vi "Resize Rendez-Vous.vi"(8 "error in (no error)":errorcluster, 10 "Resize":i32, 11 "SMO":refnum<class "SMO.lvclass">) -> (0 "error out":errorcluster, 3 "SMO out":refnum<class "SMO.lvclass">)   [LabVIEW 2013, in "SMO.lvclass"]
uses:
  SMO.lvclass
  SMO.lvclass/SMO.ctl
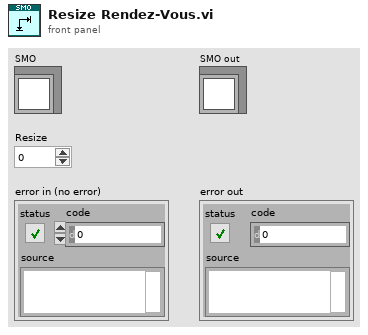
[diagram p1: front panel]
types:
  T1 = typedef "SMO.lvclass/PrivateData--Ref.ctl" = refnum<data-value>
  T2 = typedef "SMO.lvclass/PrivateData--Cluster.ctl" = cluster{"SMO Name":string, "Parent Call":T3, "Registered Processes":T4[], "Process Sync RendezVous":T5, "Process Error Notifier":refnum<notifier>, "Protected Events":T6, "Public Events":T7}
  T3 = typedef "SMO.lvclass/Parent Call--Enum.ctl" = enum16{"Allows parent to run", "Does not request parent to run"}
  T4 = typedef "SMO.lvclass/RegisteredProcessData--Cluster.ctl" = cluster{"Name":string, "Static VI Ref":refnum<vi>, "Running":bool}
  T5 = typedef "Rendezvous RefNum" = refnum<k1>
  T6 = typedef "SMO.lvclass/Protected Events.ctl" = cluster{"StopProcesses":refnum<user-event>, "AbortProcesses":refnum<user-event>}
  T7 = typedef "SMO.lvclass/Public Events.ctl" = cluster{"Error":refnum<user-event>}
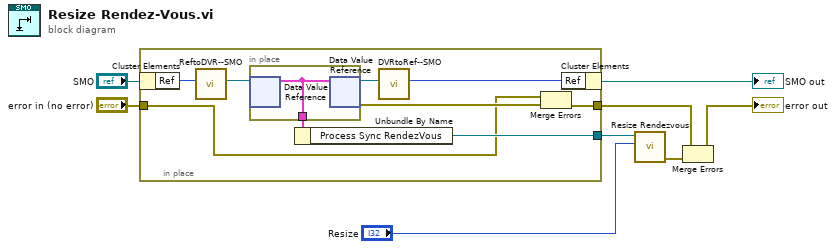
[diagram p0: block diagram]
diagram:
  n1 = in-place {
    in-place-border: [w15] -> w3
    in-place-border: [w10] -> w6
    in-place-border: "error in (no error)" -> [w9]
    n2 = in-place-cluster #1("SMO") -> ("Ref"=w14:u32)
    n3 = call "ReftoDVR--SMO.vi"("Ref"=w14) -> ("Ref"=w13:T1)  [unwired: 10 in]
    n4 = in-place {
      in-place-border: [w18] -> w17
      n5 = in-place-dvr #2(w13) -> (w18:T2)  [unwired: 1 out]
      n6 = in-place-dvr #2(w18) -> (w12:T1, w16:errorcluster)
    }
    n7 = Unbundle By Name(w17) -> ("Process Sync RendezVous"=w10:T5)
    n8 = call "DVRtoRef--SMO.vi"("Ref"=w12) -> ("Ref"=w11:u32)  [unwired: 10 in]
    n9 = Merge Errors(w9, w16) -> (w15:errorcluster)
    n10 = in-place-cluster #1("Ref"=w11) -> (→"SMO out":refnum<class "SMO.lvclass">)
  }
  n11 = call <vilib>:"Resize Rendezvous.vi"("size change (0)"="Resize", "rendezvous"=w6) -> ("error out"=w5:errorcluster)  [unwired: 3 in, 2 out]
  n12 = Merge Errors(w3, w5) -> (→"error out":errorcluster)
